vi "com port select v1.vi"(8 "error in (no error)":errorcluster, 9 "Ctl Refnum":refnum<vi>, 11 "VISA resource name in":refnum<visa-resource-name>) -> (0 "error out":errorcluster, 1 "COM PORT?":bool, 3 "VISA resource name out":refnum<visa-resource-name>)   [LabVIEW 2016]
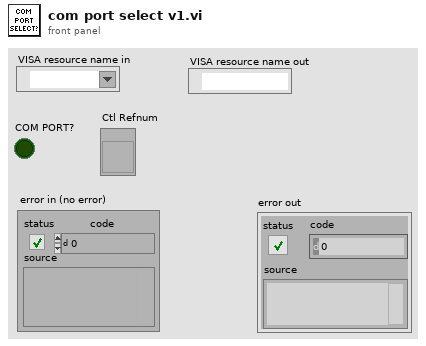
[diagram p1: front panel]
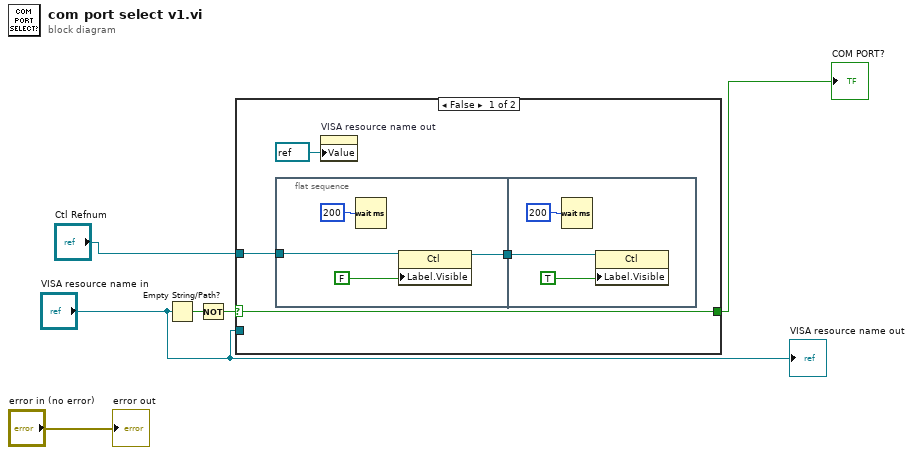
[diagram p0: block diagram]
diagram:
  n1 = Empty String/Path?(string/path="VISA resource name in") -> (empty?=w3:bool)
  n2 = Not(x=w3) -> (.not. x?=w2:bool)
  n3 = case shown="False" w2 {
    selector: w2 -> [w9 w18]
    tunnel: "VISA resource name in" -> [_ _]
    tunnel: [w9 w18] -> w4
    tunnel: "Ctl Refnum" -> [w8 _]
    frame False {
      n4 = flat-sequence {
        tunnel: w8 -> [w13]
        tunnel: [w11] -> w7
        tunnel: w7 -> [w16]
        frame #0 {
          n5 = Wait (ms)(milliseconds to wait=u32 200) -> ()  [unwired: 1 out]
          n6 = property class="Ctl"(reference=w13, "Label.Visible"=FALSE) -> (reference out=w11:refnum<vi>)  [unwired: 1 in, 1 out]
        }
        frame #1 {
          n7 = Wait (ms)(milliseconds to wait=u32 200) -> ()  [unwired: 1 out]
          n8 = property class="Ctl"(reference=w16, "Label.Visible"=TRUE) -> ()  [unwired: 1 in, 2 out]
        }
      }
      n9 = property on="VISA resource name out" class="VISAName"("Value"=refnum<visa-resource-name> refnum ("VISA resource name 2")) -> ()  [unwired: 2 in, 2 out]
    }
    frame True {
    }
  }
  "COM PORT?" <- w4
  "VISA resource name out" <- "VISA resource name in"
  "error out" <- "error in (no error)"
